vi "Blend.vi"(7 "Source Name in":string, 8 "error in (no error)":errorcluster, 9 "Source Enqueuer":refnum<class "Message Enqueuer.lvclass">, 10 "Sample to Blend in":refnum<class "Sample.lvclass">, 11 "Syringe Line in":refnum<class "Syringe Line.lvclass">) -> (0 "error out":errorcluster, 2 "Source Name":string, 3 "Syringe Line out":refnum<class "Syringe Line.lvclass">)   [LabVIEW 2015, in "cRIO-Carbondioxide.lvlib" / "CO2-Actor.lvlib" / "Syringe Line.lvclass"]
uses:
  Syringe Line.lvclass
  subs/Sample/Sample.lvclass
  <vilib>/ActorFramework/Message Enqueuer/Message Enqueuer.lvclass
  <vilib>/Utility/error.llb/Error Cluster From Error Code.vi
  CO2 Actor/CO2 Actor.lvclass
  <vilib>/ErrorRing/Error Ring.xnode
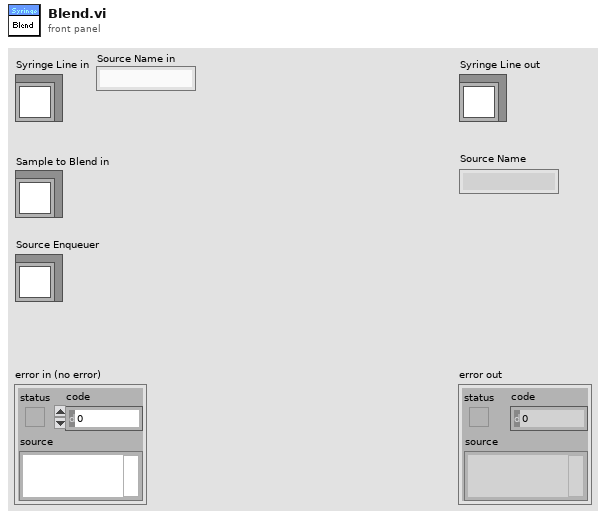
[diagram p1: front panel]
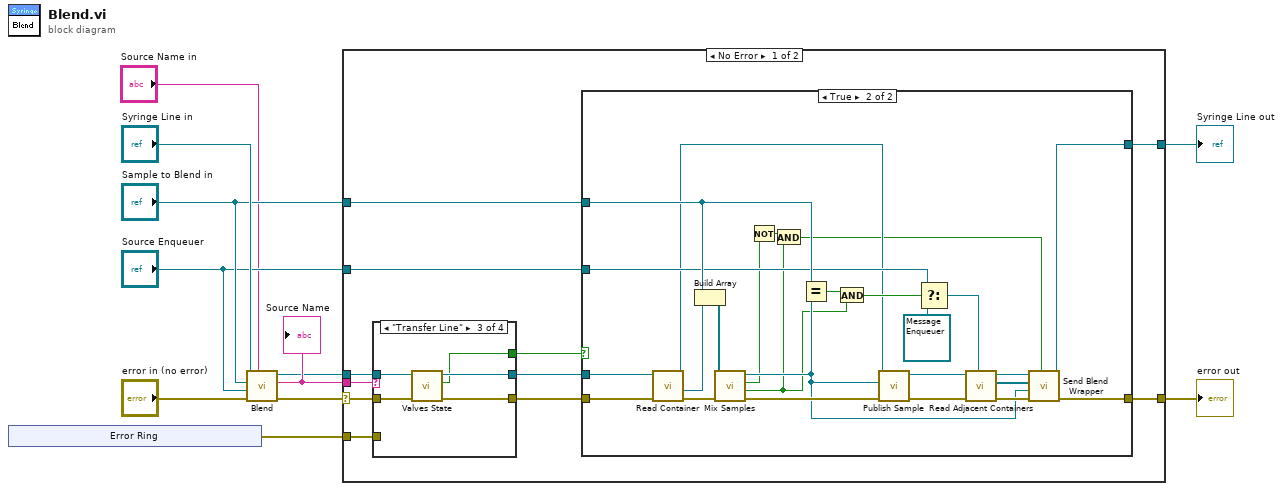
[diagram p0: block diagram]
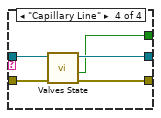
[diagram p5: hidden frame]
diagram:
  n1 = xnode "Error Ring"() -> ("error out"=w2:errorcluster)
  n2 = call-parent "Blend.vi"("Source Name in"="Source Name in", "error in (no error)"="error in (no error)", "Source Enqueuer"="Source Enqueuer", "Sample to Blend in"="Sample to Blend in", "CO2 Actor in"="Syringe Line in") -> ("error out"=w9:errorcluster, "Source Name"=w4:string, "CO2 Actor out"=w3:refnum<class "Syringe Line.lvclass">)  [unwired: 4 in]
  "Source Name" <- w4
  n3 = case shown="No Error" w9 {
    selector: w9 -> [w17 w65]
    tunnel: [w19 w65] -> w8
    tunnel: [w22 w64] -> w7
    tunnel: "Sample to Blend in" -> [w21 _]
    tunnel: "Source Enqueuer" -> [w20 _]
    tunnel: w4 -> [w18 _]
    tunnel: w3 -> [w14 w64]
    tunnel: w2 -> [w13 _]
    frame No Error {
      n4 = case shown="\"Transfer Line\"" w18 {
        tunnel: w17 -> [_ w52 w58 w63]
        tunnel: [w50 w52 w57 w62] -> w16
        tunnel: [w51 w53 w55 w61] -> w15
        tunnel: w14 -> [w51 w53 w56 w60]
        tunnel: [_ _ w54 w59] -> w12
        tunnel: w13 -> [w50 _ _ _]
        frame "False", Default {
        }
        frame "" {
        }
        frame "Transfer Line" {
          n5 = call "Valves State.vi"("error in (no error)"=w58, "Syringe in"=w56) -> ("error out"=w57:errorcluster, "Valve Transfer Line Open"=w54:bool, "Syringe out"=w55:refnum<class "Syringe Line.lvclass">)  [unwired: 6 in, 1 out]
        }
        frame "Capillary Line" {
          n6 = call "Valves State.vi"("error in (no error)"=w63, "Syringe in"=w60) -> ("error out"=w62:errorcluster, "Valve Capillar Open"=w59:bool, "Syringe out"=w61:refnum<class "Syringe Line.lvclass">)  [unwired: 6 in, 1 out]
        }
      }
      n7 = case shown="True" w12 {
        tunnel: [w24 w49] -> w22
        tunnel: w21 -> [_ w48]
        tunnel: w20 -> [_ w47]
        tunnel: [w23 w46] -> w19
        tunnel: w16 -> [w23 w26]
        tunnel: w15 -> [w24 w25]
        frame False {
        }
        frame True {
          n8 = call "Read Container.vi"("error in (no error)"=w26, "Syringe Line in"=w25) -> ("error out"=w45:errorcluster, "Sample"=w43:refnum<class "Sample.lvclass">, "Syringe Line out"=w31:refnum<class "Syringe Line.lvclass">)  [unwired: 6 in, 1 out]
          n9 = Build Array(w48, w43) -> (w44:refnum<class "Sample.lvclass">[])
          n10 = call "Mix Samples.vi"("error in (no error)"=w45, "Samples In"=w44) -> ("error out"=w42:errorcluster, "is clean?"=w30:bool, "Empty Samples present?"=w29:bool, "Sample out"=w33:refnum<class "Sample.lvclass">)  [unwired: 6 in]
          n11 = Not(x=w29) -> (.not. x?=w28:bool)
          n12 = And(x=w28, y=w30) -> (x .and. y?=w27:bool)
          n13 = Equal?(x=w48, y=w33) -> (x = y?=w39:bool)
          n14 = And(x=w39, y=w30) -> (x .and. y?=w38:bool)
          n15 = call "Publish Sample.vi"("error in (no error)"=w42, "Sample"=w33, "Syringe Line in"=w31) -> ("error out"=w41:errorcluster, "Syringe Line out"=w40:refnum<class "Syringe Line.lvclass">)  [unwired: 7 in]
          n16 = Select(t=w47, s=w38, f=refnum<class "Message Enqueuer.lvclass"> refnum) -> (s? t:f=w36:refnum<class "Message Enqueuer.lvclass">)
          n17 = call "Read Adjacent Containers.vi"("Exclude Source"=w36, "error in (no error)"=w41, "Syringe Line in"=w40) -> ("error out"=w35:errorcluster, "Adjacent Containers"=w32:refnum<class "Message Enqueuer.lvclass">[], "Syringe Line out"=w34:refnum<class "Syringe Line.lvclass">)  [unwired: 6 in]
          n18 = call-dynamic "Send Blend Wrapper.vi"("Include Source EnQr (T)"=w27, "error in (no error)"=w35, "Sample to Blend"=w33, "Send to"=w32, "CO2 Actor in"=w34) -> ("error out"=w46:errorcluster, "CO2 Actor out"=w49:refnum<class "Syringe Line.lvclass">)  [unwired: 5 in]
        }
      }
    }
    frame Error {
    }
  }
  "error out" <- w8
  "Syringe Line out" <- w7
